vi "PrefDialog.vi"(8 "error in (no error)":errorcluster, 11 "MyPluginsBase in":refnum<class "NHRDCPower.lvclass">) -> (0 "error out":errorcluster, 1 "Save As":bool, 2 "Changed":bool, 3 "MyPluginsBase out":refnum<class "NHRDCPower.lvclass">)   [LabVIEW 2018, in "AcPwrPlugins.lvlib" / "NHRDCPower.lvclass"]
doc: "This VI displays the prior instruments properties and allows a user to change the instrument properties and save these new set properties to the same location on disk or in a new location with a new name called \"Type\"."
uses:
  NHRDCPower.lvclass
  C:/Users/ico/Documents/Projects/NistPluggableModules/AcPwr/AcPwrPlugins/AcPwrBaseClass/AcPwrBase.lvclass
  C:/Program Files (x86)/National Instruments/LabVIEW 2018/user.lib/NIST/BaseClasses/BasePlugin_class/BasePlugin.lvclass
  TypeDefs/Device(s)Settings.ctl
  TypeDefs/Measurements.ctl
  AcPwrBaseClass/AcPwrBase.lvclass/AcPwrBase.ctl
  <userlib>/NIST/BaseClasses/BasePlugin_class/BasePlugin.lvclass/BasePlugin.ctl
  AcPwrBaseClass/Accessors/Read RefreshTime.vi
  <userlib>/NIST/BaseClasses/BasePlugin_class/Accessors/Read PluginIniFilePath.vi
  AcPwrBaseClass/Accessors/Write RefreshTime.vi
  <userlib>/NIST/BaseClasses/BasePlugin_class/Accessors/Write PluginIniFilePath.vi
  <vilib>/Utility/config.llb/NI_LVConfig.lvlib
  AcPwrBaseClass/AcPwrBase.lvclass
panel:
  in  "Measurements":T1 {"Fetch Method" items=["Aperture", "Immediate"]; "Measurement" items=["Voltage"=1, "Positive Peak Voltage"=2, "Positive Peak Voltage Last Fetch"=4, "Negative Peak Voltage"=8, "Negative Peak Voltage Last Fetch"=16, "Current"=32, "Positive Peak Current"=64, "Positive Peak Current Last Fetch"=128, "Negative Peak Current"=256, "Negative Peak Current Last Fetch"=512, "Power"=1024, "Positive Peak Power"=2048, "Positive Peak Power Last Fetch"=4096, "Negative Peak Power"=8192, "Negative Peak Power Last Fetch"=16384, "Timestamp"=32768, "Charge Time"=65536, "Discharge Time"=131072, "Amp Hour"=262144, "Amp Hour Time"=524288, "Amp Hour Charge"=1048576, "Amp Hour Discharge"=2097152, "Kilo Watt Hour"=4194304, "Kilo Watt Hour Time"=8388608, "Kilo Watt Hour Charge"=16777216, "Kilo Watt Hour Discharge"=33554432, "UUT Temperature"=67108864]}
  in  "Device(s)Settings":T2 {"OutputSettings"."operating state (Off)" items=["Off", "Stand By", "Charge", "Discharge", "Battery Emulation"]; "Phase Select" items=["Phase ALL", "Phase A", "Phase B", "Phase C"]}
  in  "btnSaveAs":bool
  in  "btnSave":bool
  in  "Measurement RefreshTime (s)":dbl
  in  "btnCancel":bool
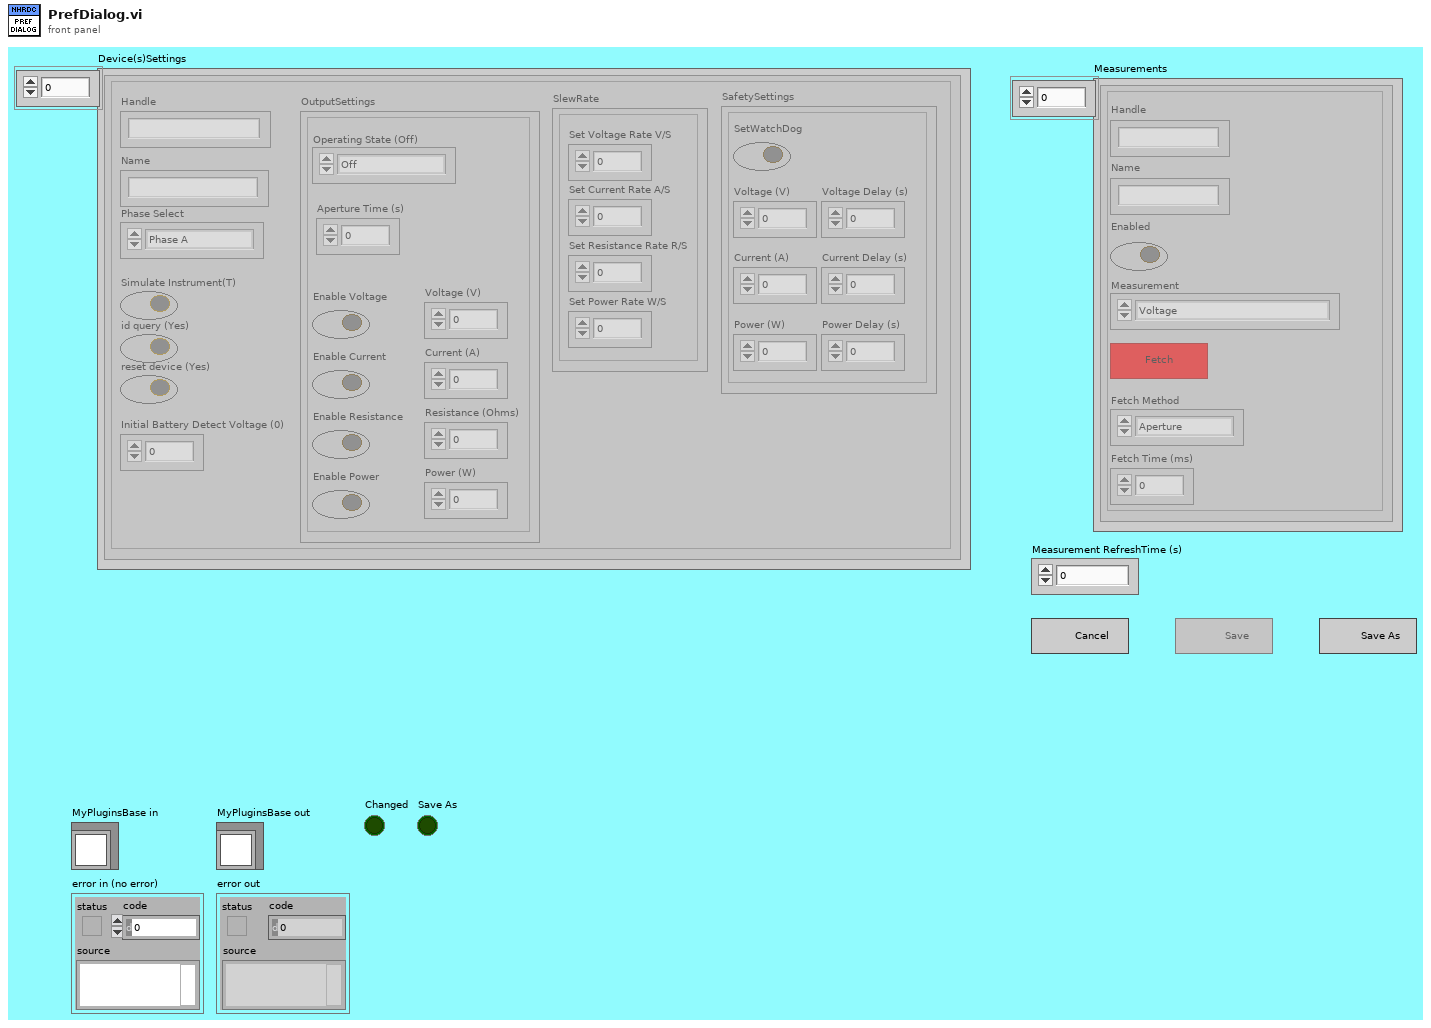
[diagram p1: front panel]
types:
  T1 = typedef "AcPwrPlugins.lvlib/NHRDCPower.lvclass/Measurements.ctl" = cluster{"Handle":string, "Name":string, "Enabled":bool, "Measurement Value":sgl, "btnMeasFetch":bool, "Measurement":i32, "Fetch Method":i32, "Fetch Time (ms)":i32}[]
  T2 = typedef "AcPwrPlugins.lvlib/NHRDCPower.lvclass/Device(s)Settings.ctl" = cluster{"Handle":string, "Name":string, "Phase Select":i32, "id query (Yes)":bool, "reset device (Yes)":bool, "Connected":bool, "Voltage Range (V)":dbl[], "Timing":cluster{"TimingOn":enum16{""}, "Hours":u32, "Minutes":u32, "Seconds":dbl, "CutoffVoltage":dbl}, "Simulate Instrument(T)":bool, "SlewRate":cluster{"Set Voltage Rate V/S":sgl, "Set Current Rate A/S":sgl, "Set Resistance Rate R/S":sgl, "Set Power Rate W/S":sgl}, "OutputSettings":cluster{"operating state (Off)":i32, "Voltage (V)":sgl, "Current (A)":sgl, "Resistance (Ohms)":sgl, "Power (W)":sgl, "Enable Voltage":bool, "Enable Current":bool, "Enable Resistance":bool, "Enable Power":bool, "Aperture Time (s)":sgl}, "Initial Battery Detect Voltage (0)":dbl, "SafetySettings":cluster{"SetWatchDog":bool, "Voltage (V)":sgl, "Current (A)":sgl, "Power (W)":sgl, "Voltage Delay (s)":sgl, "Current Delay (s)":sgl, "Power Delay (s)":sgl}}[]
  T3 = enum8{"Enabled", "Disabled", "Disabled and Grayed Out"}
  T4 = enum32{"Invalid", "Standard", "Closed", "Hidden", "Minimized", "Maximized"}
  T5 = enum32{"Invalid", "Default", "Floating", "Floating/Auto-Hide", "Modal"}
  T6 = cluster{"Handle":string, "Name":string, "Phase Select":i32, "id query (Yes)":bool, "reset device (Yes)":bool, "Connected":bool, "Voltage Range (V)":dbl[], "Timing":cluster{"TimingOn":enum16{""}, "Hours":u32, "Minutes":u32, "Seconds":dbl, "CutoffVoltage":dbl}, "Simulate Instrument(T)":bool, "SlewRate":cluster{"Set Voltage Rate V/S":sgl, "Set Current Rate A/S":sgl, "Set Resistance Rate R/S":sgl, "Set Power Rate W/S":sgl}, "OutputSettings":cluster{"operating state (Off)":i32, "Voltage (V)":sgl, "Current (A)":sgl, "Resistance (Ohms)":sgl, "Power (W)":sgl, "Enable Voltage":bool, "Enable Current":bool, "Enable Resistance":bool, "Enable Power":bool, "Aperture Time (s)":sgl}, "Initial Battery Detect Voltage (0)":dbl, "SafetySettings":cluster{"SetWatchDog":bool, "Voltage (V)":sgl, "Current (A)":sgl, "Power (W)":sgl, "Voltage Delay (s)":sgl, "Current Delay (s)":sgl, "Power Delay (s)":sgl}}
  T7 = typedef "NI_LVConfig.lvlib/Config Data RefNum.ctl" = refnum<k1>
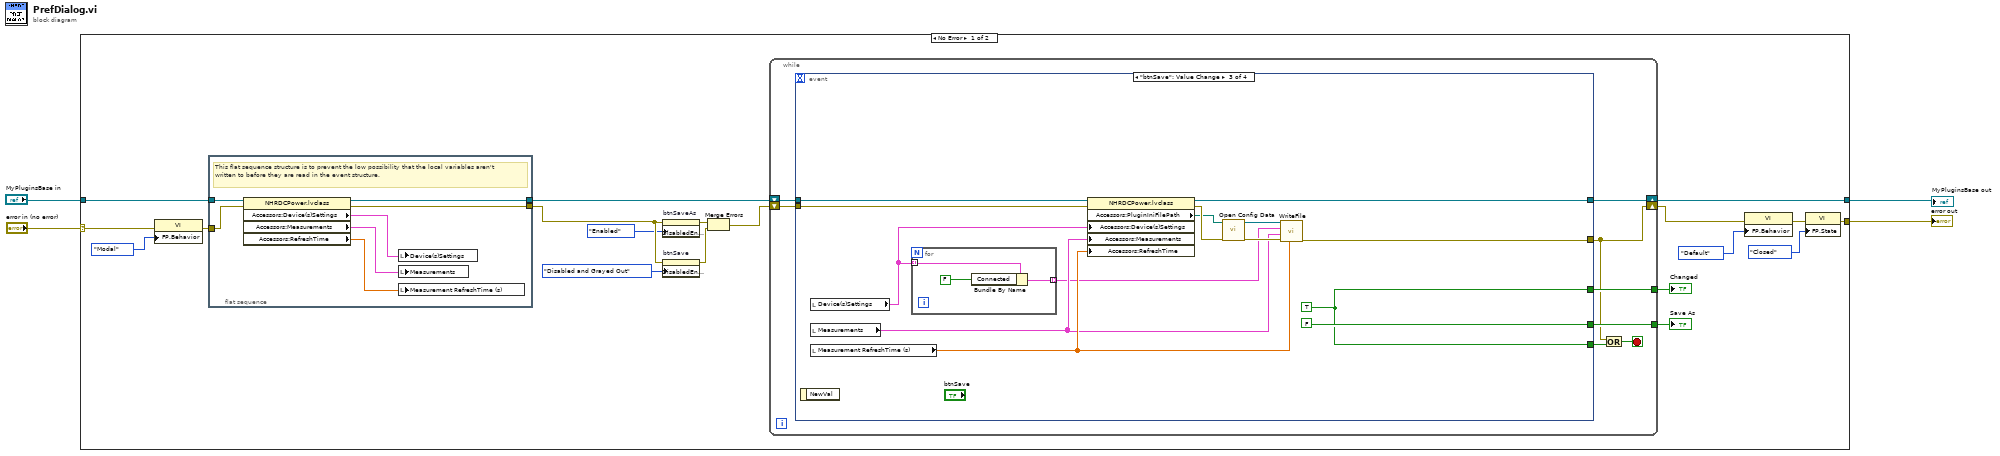
[diagram p0: block diagram]
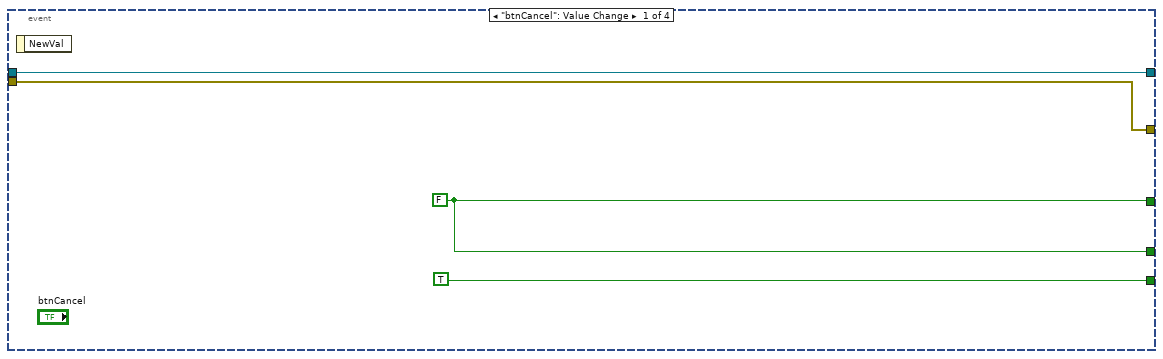
[diagram p2: hidden frame]
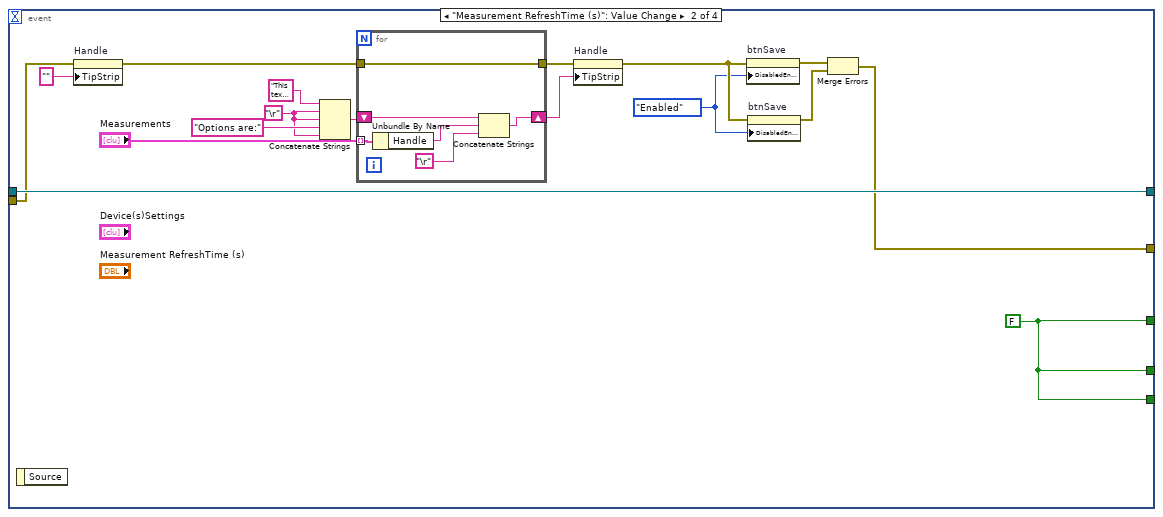
[diagram p3: hidden frame]
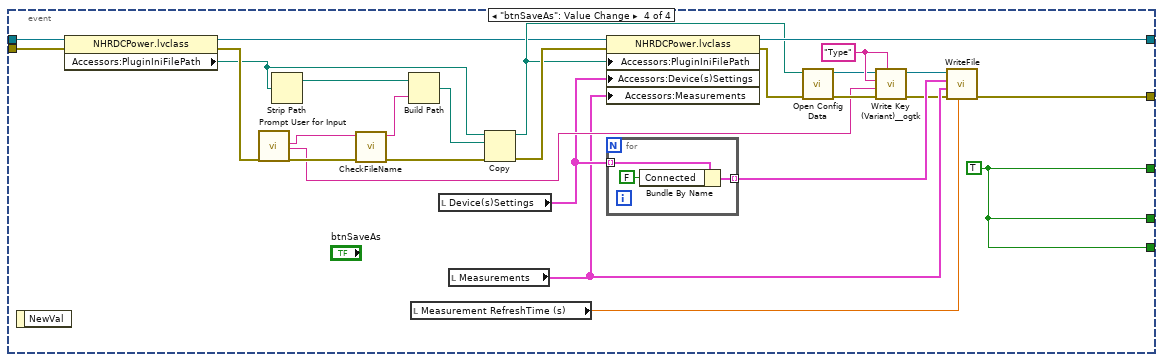
[diagram p4: hidden frame]
diagram:
  n1 = case shown="No Error" "error in (no error)" {
    selector: "error in (no error)" -> [w22 w114]
    tunnel: "MyPluginsBase in" -> [w17 w113]
    tunnel: [w15 w113] -> w2
    tunnel: [w14 w114] -> w1
    frame No Error {
      n2 = property class="VI"(error in=w22, "FP.Behavior"=T5."Modal" ("Front Panel Window:Behavior")) -> (error out=w18:errorcluster)  [unwired: 1 in, 1 out]
      n3 = flat-sequence {
        tunnel: w17 -> [w30]
        tunnel: [w29] -> w16
        tunnel: [w27] -> w12
        tunnel: w18 -> [w28]
        frame #0 {
          # "This flat sequence structure is to prevent the low possibility that the local variables aren't written to before they are read in the event structure."
          n4 = property class="NHRDCPower.lvclass"(reference=w30, error in=w28) -> (reference out=w29:refnum<class "NHRDCPower.lvclass">, error out=w27:errorcluster, "Accessors:Device(s)Settings"=w24:T2, "Accessors:Measurements"=w25:T1, "Accessors:RefreshTime"=w26:dbl)
          n5 = local write "Device(s)Settings"(w24) -> ()
          n6 = local write "Measurements"(w25) -> ()
          n7 = local write "Measurement RefreshTime (s)"(w26) -> ()
        }
      }
      n8 = property on="btnSaveAs" class="Bool"(error in=w12, "DisabledEnum"=T3."Enabled" ("Disabled")) -> (error out=w8:errorcluster)  [unwired: 1 in, 1 out]
      n9 = property on="btnSave" class="Bool"(error in=w12, "DisabledEnum"=T3."Disabled and Grayed Out" ("Disabled")) -> (error out=w7:errorcluster)  [unwired: 1 in, 1 out]
      n10 = Merge Errors(w8, w7) -> (w11:errorcluster)
      n11 = while {
        shift-right: [w35] -> w15
        shift-left: w16 -> [w36]
        tunnel: [w38] -> w10
        tunnel: [w33] -> w9
        shift-right: [w31] -> w13
        shift-left: w11 -> [w34]
        stop <- w32 stop-if-true
        n12 = event shown="[2] \"btnSave\": Value Change" {
          selector: _ -> [_ _ _ _]
          dyn-events: _ -> [_ _ _ _]
          timeout: _ -> [_ _ _ _]
          tunnel: [w39 w58 w75 w105] -> w38
          tunnel: [TRUE w58 w75 w105] -> w37
          tunnel: w36 -> [w41 w59 w78 w95]
          tunnel: [w41 w59 w74 w109] -> w35
          tunnel: [w40 w57 w71 w84] -> w31
          tunnel: w34 -> [w40 w43 w77 w94]
          tunnel: [w39 w58 FALSE w105] -> w33
          event "btnCancel": Value Change {
            w39 = FALSE
            n13 = event-data() -> ()  [unwired: 1 in, 1 out]
          }
          event "Measurement RefreshTime (s)": Value Change {
            w44 = T3."Enabled" ("Disabled")
            w54 = "\r"
            w58 = FALSE
            n14 = event-data() -> ()  [unwired: 1 in, 1 out]
            n15 = property on="Handle" class="Str"(error in=w43, "TipStrip"="" ("Tip Strip")) -> (error out=w49:errorcluster)  [unwired: 1 in, 1 out]
            n16 = Concatenate Strings("This text in this handle of the instrument and entered in the  \nhandle control in the Phases array EXACTLY, lest the attempt \nto interact with the instrument will fail.", w54, w54, "Options are:" ("Handle"), w54) -> (w53:string)
            n17 = for {
              shift-right: [w65] -> w52
              shift-left: w53 -> [w64]
              tunnel: w49 -> [w62]
              tunnel: [w62] -> w48
              tunnel: "Measurements" -> [w61] mode=indexing
              n18 = Unbundle By Name(w61) -> ("Handle"=w60:string)
              n19 = Concatenate Strings(w64, w60, "\r") -> (w65:string)
            }
            n20 = property on="Handle" class="Str"(error in=w48, "TipStrip"=w52) -> (error out=w50:errorcluster)  [unwired: 1 in, 1 out]
            n21 = property on="btnSave" class="Bool"(error in=w50, "DisabledEnum"=w44) -> (error out=w46:errorcluster)  [unwired: 1 in, 1 out]
            n22 = property on="btnSave" class="Bool"(error in=w50, "DisabledEnum"=w44) -> (error out=w45:errorcluster)  [unwired: 1 in, 1 out]
            n23 = Merge Errors(w46, w45) -> (w57:errorcluster)
          }
          event "btnSave": Value Change {
            w75 = TRUE ("StartMeas")
            n24 = event-data() -> ()  [unwired: 1 in, 1 out]
            n25 = local read "Device(s)Settings"() -> (w72:T2)
            n26 = local read "Measurements"() -> (w67:T1)
            n27 = local read "Measurement RefreshTime (s)"() -> (w68:dbl)
            n28 = for {
              tunnel: w72 -> [w82] mode=indexing
              tunnel: [w81] -> w66 mode=indexing
              n29 = Bundle By Name(cluster=w82, "Connected"=FALSE) -> (w81:T6)
            }
            n30 = property class="NHRDCPower.lvclass"(reference=w78, error in=w77, "Accessors:Device(s)Settings"=w72, "Accessors:Measurements"=w67, "Accessors:RefreshTime"=w68) -> (reference out=w74:refnum<class "NHRDCPower.lvclass">, error out=w79:errorcluster, "Accessors:PluginIniFilePath"=w73:path)
            n31 = call <vilib>:"Open Config Data.vi"("error in (no error)"=w79, "configuration file path"=w73) -> ("error out"=w69:errorcluster, "refnum"=w70:T7)  [unwired: 7 in, 1 out]
            n32 = call "WriteFile.vi"("RefreshTime"=w68, "Error In"=w69, "Measurements"=w67, "Device(s)Settings"=w66, "refnum"=w70) -> ("error out"=w71:errorcluster)  [unwired: 6 in]
          }
          event "btnSaveAs": Value Change {
            w99 = "Type" ("section (optional)")
            w105 = TRUE
            n33 = event-data() -> ()  [unwired: 1 in, 1 out]
            n34 = property class="NHRDCPower.lvclass"(reference=w95, error in=w94) -> (reference out=w92:refnum<class "NHRDCPower.lvclass">, error out=w93:errorcluster, "Accessors:PluginIniFilePath"=w89:path)
            n35 = call "Prompt User for Input"("error in (no error)"=w93) -> ("File Name"=w91:string, "PluginType"=w96:string, "error out"=w102:errorcluster)  [unwired: 15 in, 1 out]
            n36 = Strip Path(path=w89) -> (stripped path=w108:path)  [unwired: 1 out]
            n37 = call "CheckFileName.vi"("Error In"=w102, "File Name in"=w91) -> ("Error Out"=w103:errorcluster, "File Name out"=w104:string)  [unwired: 8 in]
            n38 = Build Path(base path=w108, name or relative path=w104) -> (appended path=w107:path)
            n39 = local read "Measurement RefreshTime (s)"() -> (w85:dbl)
            n40 = local read "Device(s)Settings"() -> (w90:T2)
            n41 = local read "Measurements"() -> (w87:T1)
            n42 = Copy(8:w103, 10:w107, 11:w89) -> (0:w106:errorcluster, 3:w100:path)  [unwired: 2 in, 1 out]
            n43 = property class="NHRDCPower.lvclass"(reference=w92, error in=w106, "Accessors:PluginIniFilePath"=w100, "Accessors:Device(s)Settings"=w90, "Accessors:Measurements"=w87) -> (reference out=w109:refnum<class "NHRDCPower.lvclass">, error out=w101:errorcluster)
            n44 = for {
              tunnel: w90 -> [w112] mode=indexing
              tunnel: [w111] -> w86 mode=indexing
              n45 = Bundle By Name(cluster=w112, "Connected"=FALSE) -> (w111:T6)
            }
            n46 = call <vilib>:"Open Config Data.vi"("error in (no error)"=w101, "configuration file path"=w100) -> ("error out"=w97:errorcluster, "refnum"=w98:T7)  [unwired: 7 in, 1 out]
            n47 = call <userlib>:"Write Key (Variant)__ogtk.vi"("section"=w99, "error in (no error)"=w97, "key-value"=w96, "key (optional)"=w99, "refnum"=w98) -> ("error out"=w83:errorcluster, "refnum out"=w88:T7)  [unwired: 5 in]
            n48 = call "WriteFile.vi"("RefreshTime"=w85, "Error In"=w83, "Measurements"=w87, "Device(s)Settings"=w86, "refnum"=w88) -> ("error out"=w84:errorcluster)  [unwired: 6 in]
          }
        }
        n49 = Or(x=w31, y=w37) -> (x .or. y?=w32:bool)
      }
      "Save As" <- w9
      "Changed" <- w10
      n50 = property class="VI"(error in=w13, "FP.Behavior"=T5."Default" ("Front Panel Window:Behavior")) -> (error out=w21:errorcluster)  [unwired: 1 in, 1 out]
      n51 = property class="VI"(error in=w21, "FP.State"=T4."Closed" ("Front Panel Window:State")) -> (error out=w14:errorcluster)  [unwired: 1 in, 1 out]
    }
    frame Error {
    }
  }
  "error out" <- w1
  "MyPluginsBase out" <- w2
